vi "Perform Measurements.vi"(0 "Reference values":T3, 5 "measurement configuration":T1={"Mode of operation"=enum."Perform measurement", "DUT setup time"=1.0, "Source delay"=0.005, "Aperture time"=0.005, "Nominal output voltage"=3.3, "Source pin name"="", "Source sense"=1009, "Source current limit"=25.0, "Source maximum power"=300.0, "Source start voltage"=6.0, "Source stop voltage"=20.0, "Source voltage sweep points"=4, "Use Source voltage array"=FALSE, "Source voltage array"=[], "Load pin name"="", "Load sense"=1009, "Load voltage limit range"=6.0, "Load sweep type"="Logarithmic", "Load start current"=0.1, "Load stop current"=24.0, "Load current sweep points/points per decade"=10, "Use Load current array"=FALSE, "Load current array"=[], "Pin Names for Scope"=[], "vertical range"=[], "vertical offset"=[], "probe attenuation"=[], "vertical coupling"=[], "channel enabled"=[], "input impedance"=[], "max input frequency"=[], "min sample rate"=[], "reference position"=[], "min record length"=[], "enforce realtime"=[]} {"input impedance" items=["1 mega ohm"=0, "50 ohms"=2]; "vertical coupling" items=["AC", "DC", "Ground"]; "Load sense" items=["Local"=1008, "Remote"=1009]; "Source sense" items=["Local"=1008, "Remote"=1009]}, 9 "Measurement Context":refnum<class "Measure Call Context.lvclass">, 11 "error in":errorcluster) -> (4 "Source out":refnum<k15>, 6 "Load out":refnum<k15>, 8 "Measurement Results":T7, 10 "Scope waveforms":waveform(dbl)[](array[waveform]), 15 "error out":errorcluster)   [LabVIEW 2021, in "Efficiency And Load Regulation with Pin Map.lvlib"]
uses:
  Efficiency And Load Regulation with Pin Map.lvlib
  Measurement Results.ctl
  Reference values.ctl
  <vilib>/Plug-In SDKs/Clients/Session Management V1/Session Reservation/Session Reservation.lvclass
  common/builds/PMIC Common.lvlibp/Instrument Control/Scope/TClk/Instrument Info.ctl
  common/builds/PMIC Common.lvlibp/Instrument Control/Scope Parameters.ctl
  common/builds/PMIC Common.lvlibp/1abvi3w/instr.lib/niScope/Controls/niScope vertical coupling.ctl
  <vilib>/Plug-In SDKs/Measurements/Measure Call Context/Measure Call Context.lvclass
  Measurement Configuration.ctl
  <instrlib>/niScope/Controls/niScope vertical coupling.ctl
  <vilib>/Plug-In SDKs/Sessions/niScope/Get Connections - NPin MConn.vi
  <vilib>/Plug-In SDKs/Sessions/niScope/NI Session Management niScope.lvlib
  common/builds/PMIC Common.lvlibp
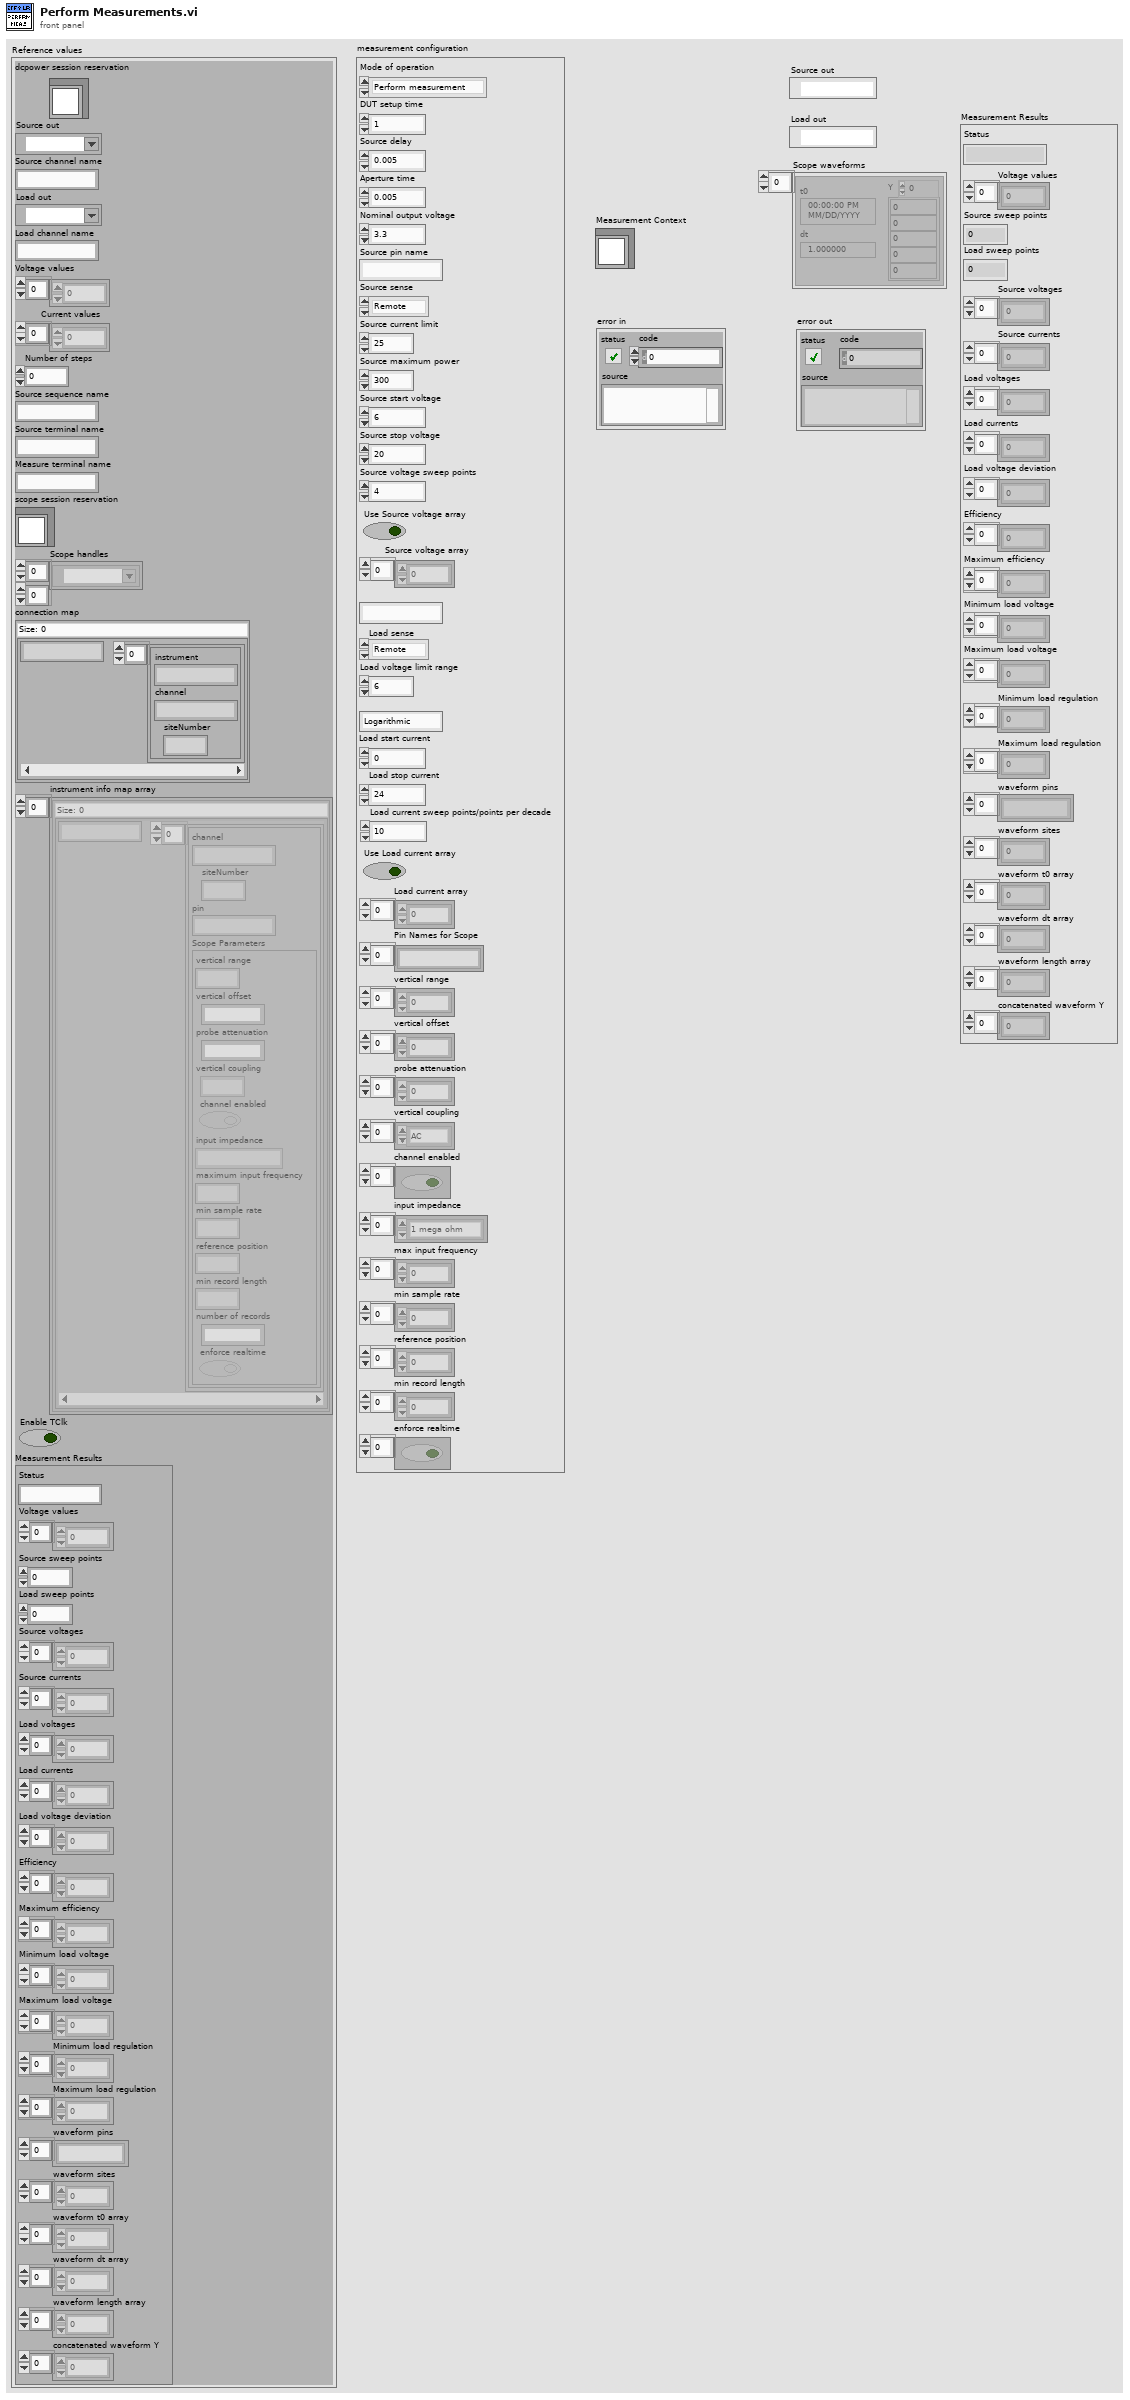
[diagram p1: front panel]
types:
  T1 = typedef "Efficiency And Load Regulation with Pin Map.lvlib/Measurement Configuration.ctl" = cluster{"Mode of operation":enum32{"Power on the DUT", "Perform measurement", "Power off the DUT"}, "DUT setup time":dbl, "Source delay":dbl, "Aperture time":dbl, "Nominal output voltage":dbl, "Source pin name":string, "Source sense":i32, "Source current limit":dbl, "Source maximum power":dbl, "Source start voltage":dbl, "Source stop voltage":dbl, "Source voltage sweep points":i32, "Use Source voltage array":bool, "Source voltage array":dbl[], "Load pin name":string, "Load sense":i32, "Load voltage limit range":dbl, "Load sweep type":string, "Load start current":dbl, "Load stop current":dbl, "Load current sweep points/points per decade":i32, "Use Load current array":bool, "Load current array":dbl[], "Pin Names for Scope":string[], "vertical range":dbl[], "vertical offset":dbl[], "probe attenuation":dbl[], "vertical coupling":T2[], "channel enabled":bool[], "input impedance":u32[], "max input frequency":dbl[], "min sample rate":dbl[], "reference position":dbl[], "min record length":i32[], "enforce realtime":bool[]}
  T2 = typedef "niScope vertical coupling.ctl" = i32
  T3 = typedef "Efficiency And Load Regulation with Pin Map.lvlib/Reference values.ctl" = cluster{"dcpower session reservation":refnum<class "Session Reservation.lvclass">, "Source out":refnum<k15>, "Source channel name":string, "Load out":refnum<k15>, "Load channel name":string, "Voltage values":dbl[], "Current values":dbl[], "Number of steps":i32, "Source sequence name":string, "Source terminal name":string, "Measure terminal name":string, "scope session reservation":refnum<class "Session Reservation.lvclass">, "Scope handles":refnum<k15>[][], "connection map":map{string, T4[]}, "instrument info map array":map{string, cluster{"channel":string, "siteNumber":i32, "pin":string, "Scope Parameters":T5}[]}[], "Enable TClk":bool, "Measurement Results":T7}
  T4 = typedef "PMIC Common.lvlibp/Instrument Info.ctl" = cluster{"instrument":string, "channel":string, "siteNumber":i32}
  T5 = typedef "PMIC Common.lvlibp/Scope Parameters.ctl" = cluster{"vertical range":dbl, "vertical offset":dbl, "probe attenuation":dbl, "vertical coupling":T6, "channel enabled":bool, "input impedance":u32, "maximum input frequency":dbl, "min sample rate":dbl, "reference position":dbl, "min record length":i32, "number of records":i32, "enforce realtime":bool}
  T6 = typedef "PMIC Common.lvlibp/niScope vertical coupling.ctl" = i32
  T7 = typedef "Efficiency And Load Regulation with Pin Map.lvlib/Measurement Results.ctl" = cluster{"Status":string, "Voltage values":dbl[], "Source sweep points":i32, "Load sweep points":i32, "Source voltages":dbl[], "Source currents":dbl[], "Load voltages":dbl[], "Load currents":dbl[], "Load voltage deviation":dbl[], "Efficiency":dbl[], "Maximum efficiency":dbl[], "Minimum load voltage":dbl[], "Maximum load voltage":dbl[], "Minimum load regulation":dbl[], "Maximum load regulation":dbl[], "waveform pins":string[], "waveform sites":i32[], "waveform t0 array":dbl[], "waveform dt array":dbl[], "waveform length array":i32[], "concatenated waveform Y":dbl[]}
  T8 = map{string, cluster{"channel":string, "siteNumber":i32, "pin":string, "Scope Parameters":T5}[]}[]
  T9 = typedef "NI Session Management niScope.lvlib/Connection with Session.ctl" = cluster{"connection":T10, "session":refnum<k15>}
  T10 = typedef "NI Session Management V1 Client.lvlib/Session Reservation.lvclass/Connection.ctl" = cluster{"pin or relay name":string, "site":i32, "instrument type id":string, "channel":string}
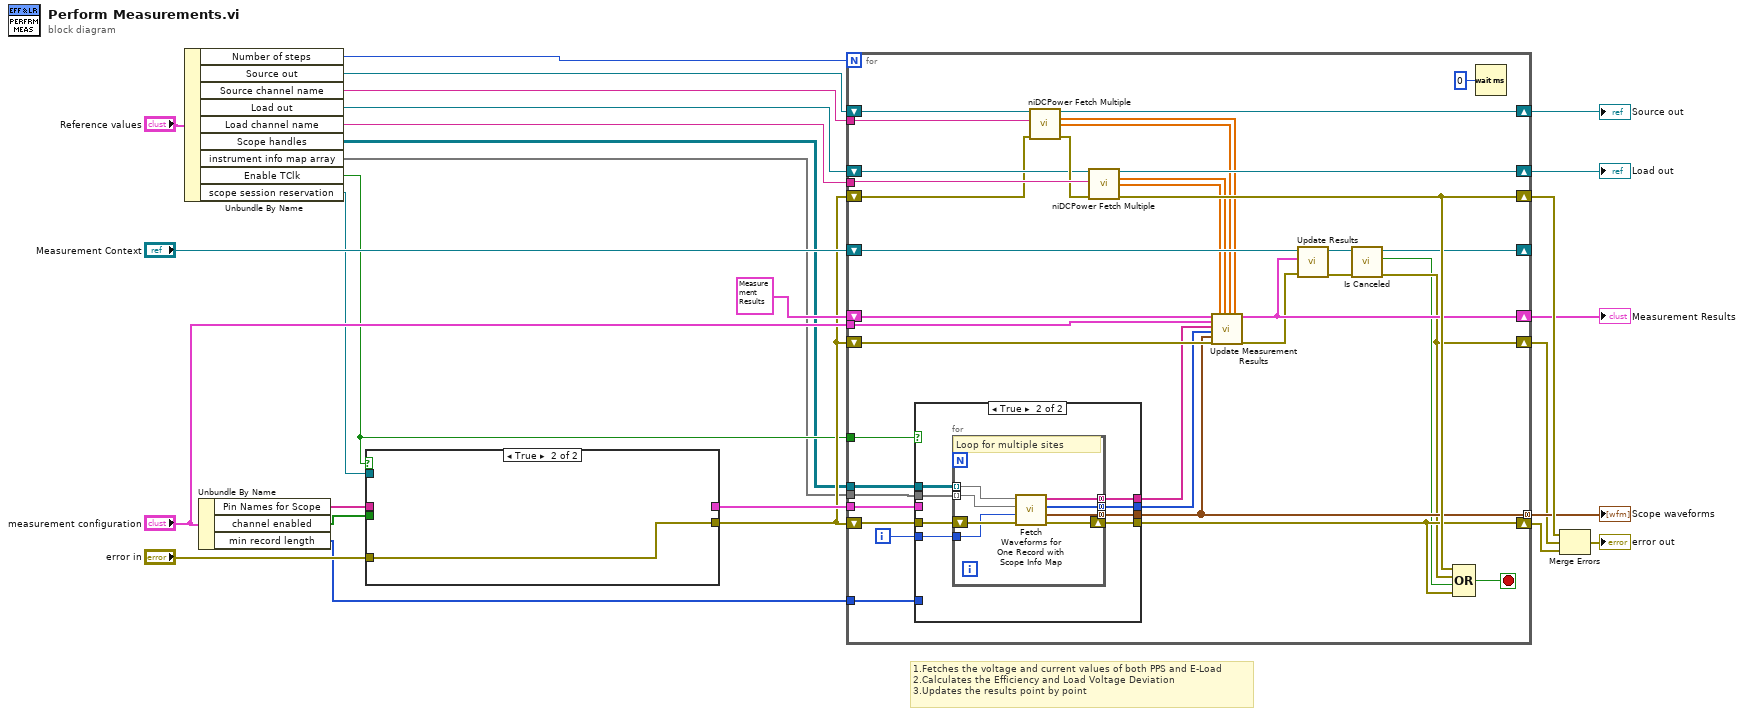
[diagram p0: block diagram]
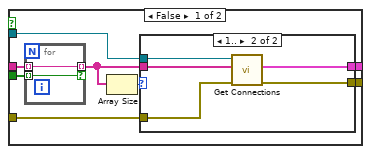
[diagram p2: hidden frame]
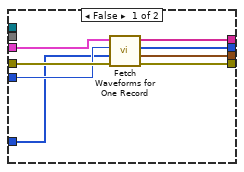
[diagram p4: hidden frame]
diagram:
  # "1.Fetches the voltage and current values of both PPS and E-Load\n2.Calculates the Efficiency and Load Voltage Deviation\n3.Updates the results point by point"
  n1 = Unbundle By Name("Reference values") -> ("Number of steps"=w8:i32, "Source out"=w23:refnum<k15>, "Source channel name"=w22:string, "Load out"=w21:refnum<k15>, "Load channel name"=w20:string, "Scope handles"=w4:refnum<k15>[][], "instrument info map array"=w3:T8, "Enable TClk"=w5:bool, "scope session reservation"=w1:refnum<class "Session Reservation.lvclass">)
  n2 = Unbundle By Name("measurement configuration") -> ("Pin Names for Scope"=w6:string[], "channel enabled"=w7:bool[], "min record length"=w2:i32[])
  n3 = case shown="True" w5 {
    tunnel: "error in" -> [w35 w44]
    tunnel: [w34 _] -> w17
    tunnel: [w33 w44] -> w11
    tunnel: w7 -> [w31 _]
    tunnel: w6 -> [w29 _]
    tunnel: w1 -> [w28 _]
    frame False {
      n4 = for {
        tunnel: w29 -> [w43] mode=indexing
        tunnel: w31 -> [w42] mode=indexing
        tunnel: [w43] -> w30 mode=indexing if=w42
      }
      n5 = Array Size(array=w30) -> (size(s)=w32:i32)
      n6 = case shown="1.." w32 {
        tunnel: w35 -> [w36 w41]
        tunnel: [_ w40] -> w34
        tunnel: w28 -> [_ w39]
        tunnel: w30 -> [_ w38]
        tunnel: [w36 w37] -> w33
        frame 0, Default {
          # "Do nothing if Pin Names are empty."
        }
        frame 1.. {
          n7 = call-poly <vilib>:"Get Connections.vi"("error in"=w41, "pin or relay names"=w38, "session reservation in"=w39) -> ("error out"=w37:errorcluster, "connections"=w40:T9[])  [unwired: 6 in, 1 out]
        }
      }
    }
    frame True {
    }
  }
  n8 = for {
    N: w8 -> [_]
    tunnel: w20 -> [w78]
    tunnel: w22 -> [w77]
    shift-right: [w79] -> w26
    shift-left: w21 -> [w75]
    shift-right: [w73] -> w27
    shift-left: w11 -> [w74]
    shift-right: [w80] -> w25
    shift-left: w23 -> [w81]
    shift-right: [w46] -> _
    shift-left: "Measurement Context" -> [w62]
    shift-right: [w66] -> w12
    shift-left: T7 {"Status"="", "Voltage values"=[], "Source sweep points"=0, "Load sweep points"=0, "Source voltages"=[], "Source currents"=[], "Load voltages"=[], "Load currents"=[], "Load voltage deviation"=[], "Efficiency"=[], "Maximum efficiency"=[], "Minimum load voltage"=[], "Maximum load voltage"=[], "Minimum load regulation"=[], "Maximum load regulation"=[], "waveform pins"=[], "waveform sites"=[], "waveform t0 array"=[], "waveform dt array"=[], "waveform length array"=[], "concatenated waveform Y"=[]} ("Measurement Results") -> [w68]
    tunnel: w17 -> [w70]
    tunnel: [w56] -> w16 mode=concatenating
    shift-right: [w64] -> w10
    shift-left: w11 -> [w69]
    tunnel: "measurement configuration" -> [w57]
    shift-right: [w47] -> w9
    shift-left: w11 -> [w63]
    tunnel: w5 -> [w55]
    tunnel: w4 -> [w54]
    tunnel: w3 -> [w53]
    tunnel: w2 -> [w50]
    i -> [w67]
    stop <- w72 stop-if-true
    n9 = case shown="True" w55 {
      tunnel: w70 -> [w84 _]
      tunnel: w69 -> [w89 w96]
      tunnel: w67 -> [w83 w93]
      tunnel: [w88 w95] -> w64
      tunnel: [w87 w94] -> w56
      tunnel: w54 -> [_ w97]
      tunnel: w53 -> [_ w92]
      tunnel: [w86 w91] -> w52
      tunnel: [w85 w90] -> w51
      tunnel: w50 -> [w82 _]
      frame False {
        n10 = call "Fetch Waveforms for One Record.vi"("error in (no error)"=w89, "min record length"=w82, "fetch record number"=w83, "connections"=w84) -> ("error out"=w88:errorcluster, "waveforms"=w87:waveform(dbl)[], "sites"=w86:i32[], "pins or relay names"=w85:string[])  [unwired: 4 in]
      }
      frame True {
        n11 = for {
          tunnel: w97 -> [w102] mode=indexing
          shift-right: [w104] -> w95
          shift-left: w96 -> [w105]
          tunnel: [w103] -> w94 mode=concatenating
          tunnel: w93 -> [w100]
          tunnel: w92 -> [w101] mode=indexing
          tunnel: [w98] -> w90 mode=concatenating
          tunnel: [w99] -> w91 mode=concatenating
          # "Loop for multiple sites"
          n12 = call "Fetch Waveforms for One Record with Scope Info Map.vi"("error in (no error)"=w105, "fetch record number"=w100, "scope info map"=w101, "Scope handles"=w102) -> ("error out"=w104:errorcluster, "waverforms"=w103:waveform(dbl)[], "sites"=w99:i32[], "pins"=w98:string[])  [unwired: 4 in]
        }
      }
    }
    n13 = call <instrlib>:"niDCPower Fetch Multiple.vi"("instrument handle"=w81, "channel name"=w77, "error in (no error)"=w74) -> ("instrument handle out"=w80:refnum<k15>, "voltage measurements"=w61:dbl[], "current measurements"=w60:dbl[], "error out"=w76:errorcluster)  [unwired: 2 in, 7 out]
    n14 = call <instrlib>:"niDCPower Fetch Multiple.vi"("instrument handle"=w75, "channel name"=w78, "error in (no error)"=w76) -> ("instrument handle out"=w79:refnum<k15>, "voltage measurements"=w59:dbl[], "current measurements"=w58:dbl[], "error out"=w73:errorcluster)  [unwired: 2 in, 7 out]
    n15 = call "Update Measurement Results.vi"("measurement results in"=w68, "measurement configuration"=w57, "waveform pins"=w51, "waveform sites"=w52, "Scope waveforms"=w56, "error in (no error)"=w63, "Load currents"=w58, "Load voltages"=w59, "Source currents"=w60, "Source voltages"=w61) -> ("measurement results out"=w66:T7, "error out"=w65:errorcluster)  [unwired: 8 in]
    n16 = call <vilib>:"Update Results.vi"("error in"=w65, "measurement results"=w66, "measure call context in"=w62) -> ("error out"=w48:errorcluster, "measure call context out"=w49:refnum<class "Measure Call Context.lvclass">)  [unwired: 7 in]
    n17 = call <vilib>:"Is Canceled.vi"("error in"=w48, "measure call context in"=w49) -> ("error out"=w47:errorcluster, "is canceled?"=w45:bool, "measure call context out"=w46:refnum<class "Measure Call Context.lvclass">)  [unwired: 7 in]
    n18 = Compound Arithmetic op=OR(w73, w47, w45, w64) -> (w72:bool)
    n19 = Wait (ms)(milliseconds to wait=u32 0) -> ()  [unwired: 1 out]
  }
  "Load out" <- w26
  "Source out" <- w25
  "Measurement Results" <- w12
  "Scope waveforms" <- w16
  n20 = Merge Errors(w27, w9, w10) -> (→"error out":errorcluster)
